vi "Unflatten BDPW.vi"(8 "error in (no error)":errorcluster, 11 "Data in":string) -> (0 "error out":errorcluster, 3 "BDPW":T1)   [LabVIEW 2021, in "VI-Hacker.lvlib"]
uses:
  VI-Hacker.lvlib
  TypeDefs/Block BDPW.ctl
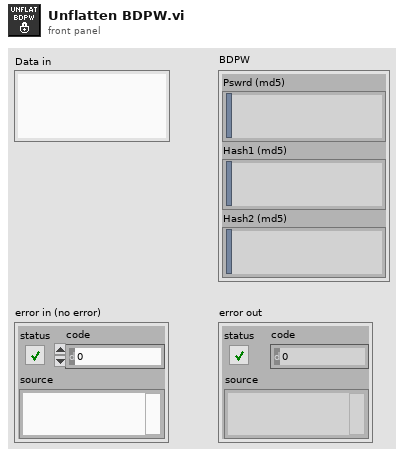
[diagram p1: front panel]
types:
  T1 = typedef "VI-Hacker.lvlib/Block BDPW.ctl" = cluster{"Pswrd (md5)":string, "Hash1 (md5)":string, "Hash2 (md5)":string}
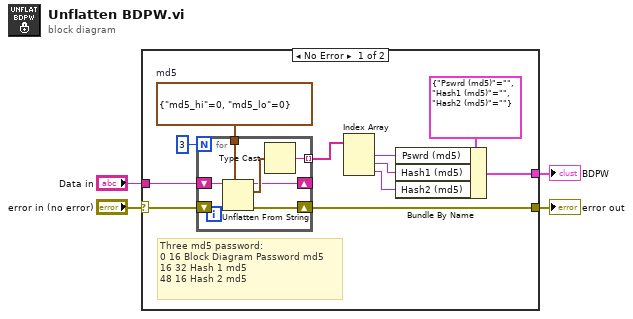
[diagram p0: block diagram]
diagram:
  n1 = case shown="No Error" "error in (no error)" {
    selector: "error in (no error)" -> [w13 w23]
    tunnel: [w15 _] -> w4
    tunnel: [w14 w23] -> w3
    tunnel: "Data in" -> [w6 _]
    frame No Error {
      w7 = cluster{"md5_hi":u64, "md5_lo":u64} {"md5_hi"=0, "md5_lo"=0}  # md5
      # "Three md5 password:\n0 16 Block Diagram Password md5\n16 32 Hash 1 md5\n48 16 Hash 2 md5"
      n2 = for {
        N: 3 -> [_]
        shift-right: [w22] -> w14
        shift-left: w13 -> [w21]
        tunnel: [w18] -> w11 mode=indexing
        shift-right: [w17] -> _
        shift-left: w6 -> [w20]
        tunnel: w7 -> [w16]
        n3 = Unflatten From String(type=w16, binary string=w20, error in (no error)=w21) -> (rest of the binary string=w17:string, value=w19:cluster{"md5_hi":u64, "md5_lo":u64}, error out=w22:errorcluster)  [unwired: 2 in]
        n4 = Type Cast(x=w19) -> (*(type *) &x=w18:string)  [unwired: 1 in]
      }
      n5 = Index Array(array=w11) -> (element #1=w10:string, element #2=w9:string, element #3=w8:string)  [unwired: 3 in]
      n6 = Bundle By Name(cluster=T1 {"Pswrd (md5)"="", "Hash1 (md5)"="", "Hash2 (md5)"=""} ("BDPW"), "Pswrd (md5)"=w10, "Hash1 (md5)"=w9, "Hash2 (md5)"=w8) -> (w15:T1)
    }
    frame Error {
    }
  }
  "error out" <- w3
  "BDPW" <- w4
